vi "hemanth.vi"() -> ()   [LabVIEW 2019]
panel:
  out "appended array":string[](array[string])
  in  "file (use dialog) 2":path
  in  "file (use dialog)":path
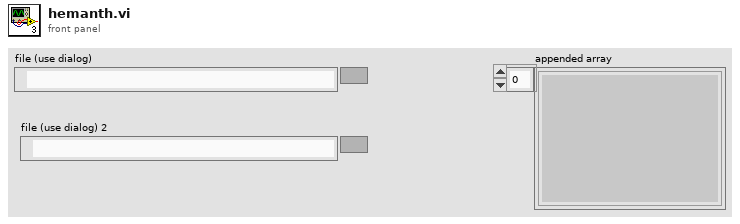
[diagram p1: front panel]
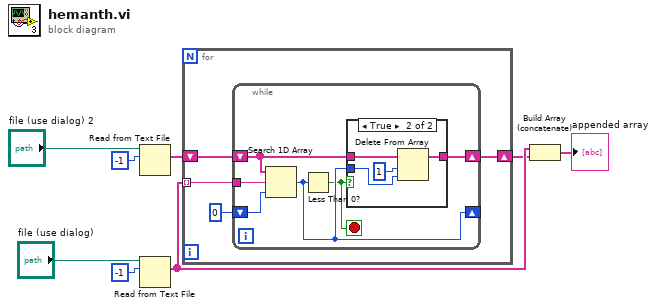
[diagram p0: block diagram]
diagram:
  n1 = Read from Text File(file (use dialog)="file (use dialog) 2", count=-1) -> (text=w4:string[])  [unwired: 2 in, 3 out]
  n2 = Read from Text File(file (use dialog)="file (use dialog)", count=-1) -> (text=w3:string[])  [unwired: 2 in, 3 out]
  n3 = for {
    tunnel: w3 -> [w12] mode=indexing
    shift-right: [w11] -> w2
    shift-left: w4 -> [w10]
    n4 = while {
      tunnel: w12 -> [w18]
      shift-right: [w17] -> w11
      shift-left: w10 -> [w16]
      shift-right: [w15] -> _
      shift-left: 0 ("index of element") -> [w14]
      stop <- w13 stop-if-true
      n5 = Search 1D Array(1D array=w16, element=w18, start index (0)=w14) -> (index of element=w15:i32)
      n6 = Less Than 0?(x=w15) -> (x < 0?=w13:bool)
      n7 = case shown="True" w13 {
        tunnel: w16 -> [w19 w23]
        tunnel: w15 -> [_ w21]
        tunnel: [w19 w20] -> w17
        frame False {
        }
        frame True {
          n8 = Delete From Array(array=w23, length=1, index=w21) -> (array with subset deleted=w20:string[])  [unwired: 1 out]
        }
      }
    }
  }
  n9 = Build Array (concatenate)(w3, w2) -> (→"appended array":string[])
